vi "Name to Icon Lines.vi"(10 "Name":string) -> (2 "Lines":string[](array[string]))   [LabVIEW 2013]
uses:
  <vilib>/regexp/Match Regular Expression.xnode
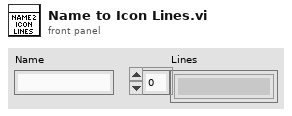
[diagram p1: front panel]
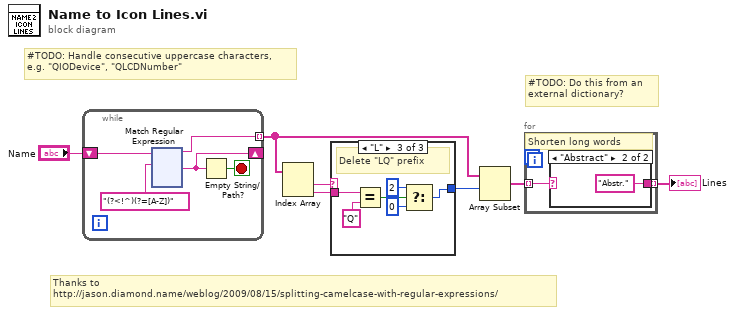
[diagram p0: block diagram]
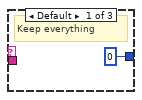
[diagram p2: hidden frame]
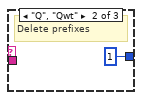
[diagram p3: hidden frame]
diagram:
  # "#TODO: Do this from an\nexternal dictionary?"
  # "#TODO: Handle consecutive uppercase characters,\ne.g. \"QIODevice\", \"QLCDNumber\""
  # "Thanks to\nhttp://jason.diamond.name/weblog/2009/08/15/splitting-camelcase-with-regular-expressions/"
  n1 = while {
    shift-right: [w9] -> _
    shift-left: "Name" -> [w10]
    tunnel: [w8] -> w2 mode=indexing
    stop <- w12 stop-if-true
    n2 = xnode "Match Regular Expression"("input string"=w10, "regular expression"="(?<!^)(?=[A-Z])") -> ("before match"=w8:string, "after match"=w9:string)  [unwired: 4 in, 3 out]
    n3 = Empty String/Path?(string/path=w9) -> (empty?=w12:bool)
  }
  n4 = Index Array(array=w2) -> (element #1=w4:string, element #2=w1:string)  [unwired: 2 in]
  n5 = case shown="\"L\"" w4 {
    tunnel: [0 ("index") 1 ("index") w129] -> w3
    tunnel: w1 -> [_ _ w134]
    frame Default {
      # "Keep everything"
    }
    frame "Q", "Qwt" {
      # "Delete prefixes"
    }
    frame "L" {
      # "Delete \"LQ\" prefix"
      n6 = Equal?(x=w134, y="Q") -> (x = y?=w132:bool)
      n7 = Select(t=2 ("index"), s=w132, f=0 ("index")) -> (s? t:f=w129:i32)
    }
  }
  n8 = Array Subset(array=w2, index=w3) -> (w6:string[])  [unwired: 1 in]
  n9 = for {
    tunnel: w6 -> [w136] mode=indexing
    tunnel: [w135] -> w5 mode=indexing
    # "Shorten long words"
    n10 = case shown="\"Abstract\"" w136 {
      selector: w136 -> [w137 _]
      tunnel: [w137 "Abstr."] -> w135
      frame Default {
      }
      frame "Abstract" {
      }
    }
  }
  "Lines" <- w5
